vi "Get Topic.vi"(8 "error in (no error)":errorcluster, 9 "Topic Type":variant, 10 "Topic Name":string, 11 "TopicLookupTable":refnum<data-value>) -> (0 "error out":errorcluster, 1 "Topic Found?":bool, 2 "Topic Refnum":refnum<class "Message Enqueuer.lvclass">, 3 "TopicLookupTable":refnum<data-value>)   [LabVIEW 2015, in "Mediator.lvlib" / "TopicLookupTable.lvclass"]
doc: "<License>\nCopyright © 2017 Composed Systems, LLC | All rights reserved\nwww.composed.io\n\nAuthor: Ethan Stern <ethan.stern@composed.io>\n\nThis software is provided \"AS IS\" WITHOUT WARRANTIES, either express or implied, AND IS FOR EDUCATIONAL PURPOSES ONLY.\n</License>"
uses:
  TopicLookupTable.lvclass
  <vilib>/ActorFramework/Message Enqueuer/Message Enqueuer.lvclass
  TopicLookupTable.lvclass/TopicLookupTable.ctl
  Topic/Topic.lvclass
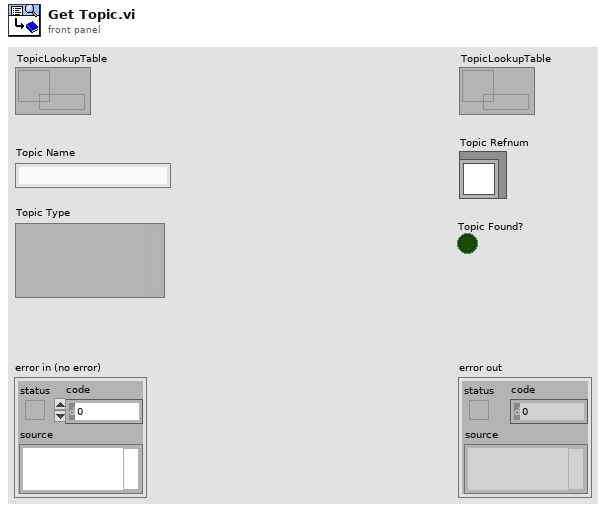
[diagram p1: front panel]
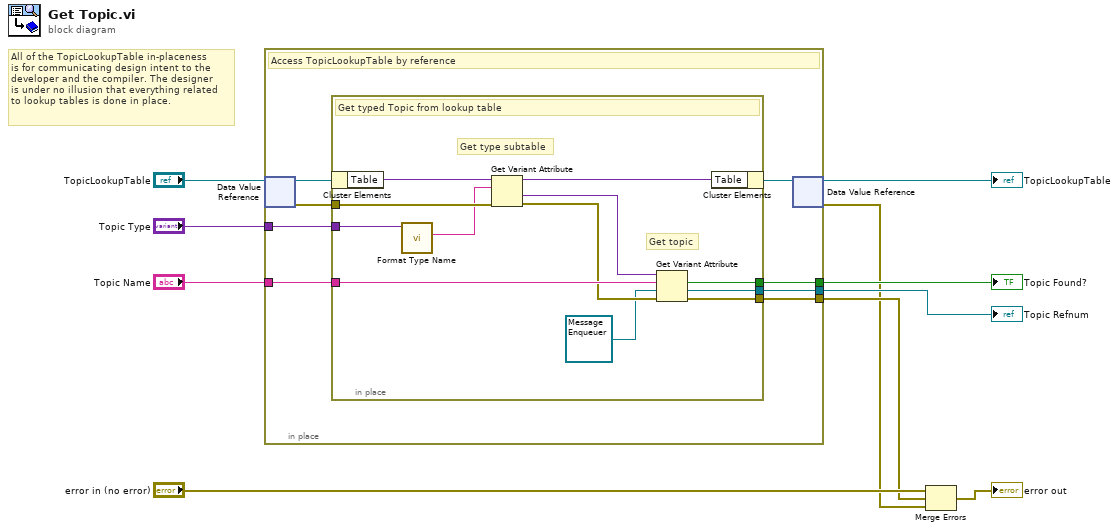
[diagram p0: block diagram]
diagram:
  # "All of the TopicLookupTable in-placeness\nis for communicating design intent to the\ndeveloper and the compiler. The designer\nis under no illusion that everything related\nto lookup tables is done in place."
  n1 = in-place {
    in-place-border: "Topic Name" -> [w18]
    in-place-border: "Topic Type" -> [w17]
    in-place-border: [w16] -> w3
    in-place-border: [w15] -> w6
    in-place-border: [w14] -> w5
    # "Access TopicLookupTable by reference"
    n2 = in-place-dvr #1("TopicLookupTable") -> (w13:refnum<class "TopicLookupTable.lvclass">, w11:errorcluster)
    n3 = in-place {
      in-place-border: w18 -> [w25]
      in-place-border: w17 -> [w24]
      in-place-border: [w23] -> w14
      in-place-border: [w22] -> w15
      in-place-border: [w20] -> w16
      in-place-border: w11 -> [w30]
      # "Get topic"
      # "Get type subtable"
      # "Get typed Topic from lookup table"
      n4 = in-place-cluster #2(w13) -> ("Table"=w29:variant)
      n5 = call "Format Type Name.vi"("Data Type"=w24) -> ("Name"=w26:string)  [unwired: 9 in, 1 out]
      n6 = Get Variant Attribute(Variant=w29, name=w26, error in=w30) -> (duplicate Variant=w27:variant, value=w28:variant, error out=w21:errorcluster)  [unwired: 1 in, 1 out]
      n7 = Get Variant Attribute(Variant=w28, name=w25, default value (empty Variant)=refnum<class "Message Enqueuer.lvclass"> refnum ("Self Enqueuer"), error in=w21) -> (found=w22:bool, value=w23:refnum<class "Message Enqueuer.lvclass">, error out=w20:errorcluster)  [unwired: 1 out]
      n8 = in-place-cluster #2("Table"=w27) -> (w12:refnum<class "TopicLookupTable.lvclass">)
    }
    n9 = in-place-dvr #1(w12) -> (→"TopicLookupTable":refnum<data-value>, w2:errorcluster)
  }
  "Topic Found?" <- w6
  "Topic Refnum" <- w5
  n10 = Merge Errors("error in (no error)", w3, w2) -> (→"error out":errorcluster)
